vi "Enqueue.vi"(0 "queue in":refnum<queue>, 1 "Priority (F)":bool, 2 "Enqueue Type (Enqueue)":T1, 5 "Message":string, 7 "Message Data":variant, 9 "MyPluginsClass":refnum<class "MyPluginsBase.lvclass">, 11 "error in (no error)":errorcluster) -> (4 "queue out":refnum<queue>, 15 "error out":errorcluster)   [LabVIEW 2018, in "MyPlugins.lvlib"]
doc: "Enqueues a message and message data based on the queue name."
uses:
  MyPlugins.lvlib
  MyPluginBaseClass/MyPluginsBase.lvclass
  QueueMessageType.ctl
  EnqueueTypes.ctl
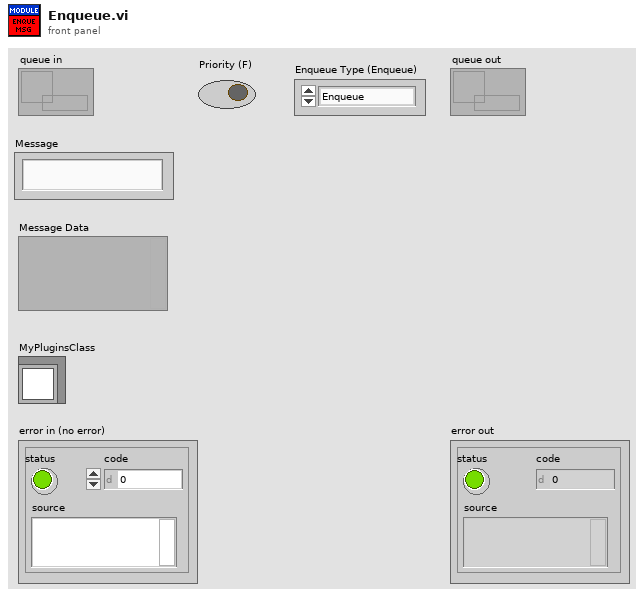
[diagram p1: front panel]
types:
  T1 = typedef "MyPlugins.lvlib/EnqueueTypes.ctl" = enum16{"Enqueue", "Lossy Enqueue"}
  T2 = typedef "MyPlugins.lvlib/QueueMessageType.ctl" = cluster{"Message":string, "Message Data":variant, "MyPluginsClass":refnum<class "MyPluginsBase.lvclass">}
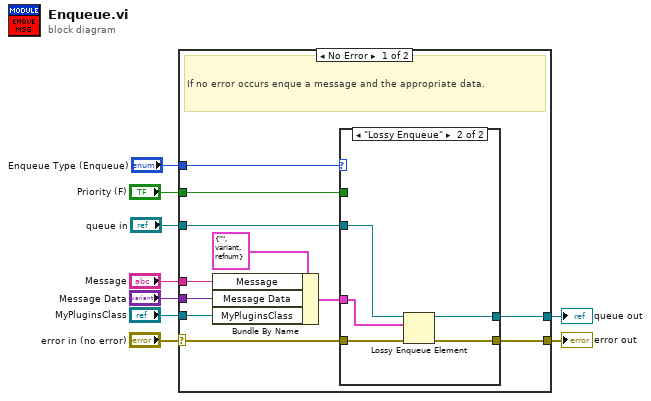
[diagram p0: block diagram]
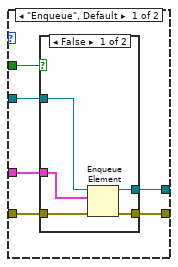
[diagram p2: hidden frame]
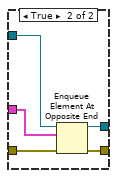
[diagram p3: hidden frame]
diagram:
  n1 = case shown="No Error" "error in (no error)" {
    selector: "error in (no error)" -> [w14 w43]
    tunnel: "Message" -> [w19 _]
    tunnel: "Message Data" -> [w18 _]
    tunnel: "Priority (F)" -> [w17 _]
    tunnel: [w16 w43] -> w5
    tunnel: "MyPluginsClass" -> [w13 _]
    tunnel: "queue in" -> [w12 w42]
    tunnel: [w11 w42] -> w2
    tunnel: "Enqueue Type (Enqueue)" -> [w10 _]
    frame No Error {
      # "If no error occurs enque a message and the appropriate data."
      n2 = Bundle By Name(cluster=T2 {"Message"="", "Message Data"=variant, "MyPluginsClass"=refnum} ("clMessage"), "Message"=w19, "Message Data"=w18, "MyPluginsClass"=w13) -> (w20:T2)
      n3 = case shown="\"Lossy Enqueue\"" w10 {
        tunnel: w20 -> [w26 w37]
        tunnel: w17 -> [w25 _]
        tunnel: [w24 w40] -> w16
        tunnel: w14 -> [w23 w41]
        tunnel: w12 -> [w22 w38]
        tunnel: [w21 w39] -> w11
        frame "Enqueue", Default {
          n4 = case shown="False" w25 {
            tunnel: w26 -> [w30 w36]
            tunnel: w22 -> [w31 w35]
            tunnel: [w29 w34] -> w24
            tunnel: w23 -> [w28 w33]
            tunnel: [w27 w32] -> w21
            frame False {
              n5 = Enqueue Element(queue=w31, element=w30, error in (no error)=w28) -> (queue out=w27:refnum<queue>, error out=w29:errorcluster)  [unwired: 1 in, 1 out]
            }
            frame True {
              n6 = Enqueue Element At Opposite End(queue=w35, element=w36, error in (no error)=w33) -> (queue out=w32:refnum<queue>, error out=w34:errorcluster)  [unwired: 1 in, 1 out]
            }
          }
        }
        frame "Lossy Enqueue" {
          n7 = Lossy Enqueue Element(queue=w38, element=w37, error in (no error)=w41) -> (queue out=w39:refnum<queue>, error out=w40:errorcluster)  [unwired: 2 out]
        }
      }
    }
    frame Error {
    }
  }
  "error out" <- w5
  "queue out" <- w2
